vi "Defocus and Spherical Comp.vi"(1 "Spherical Step":dbl, 2 "Defocus Step":dbl, 3 "Step #":i32) -> ()   [LabVIEW 2014]
uses:
  DM_Dual_V2/Controls/Standard Action.ctl
panel:
  out "Map 2":dbl[][](graph)
  out "map 1":dbl[][](graph)
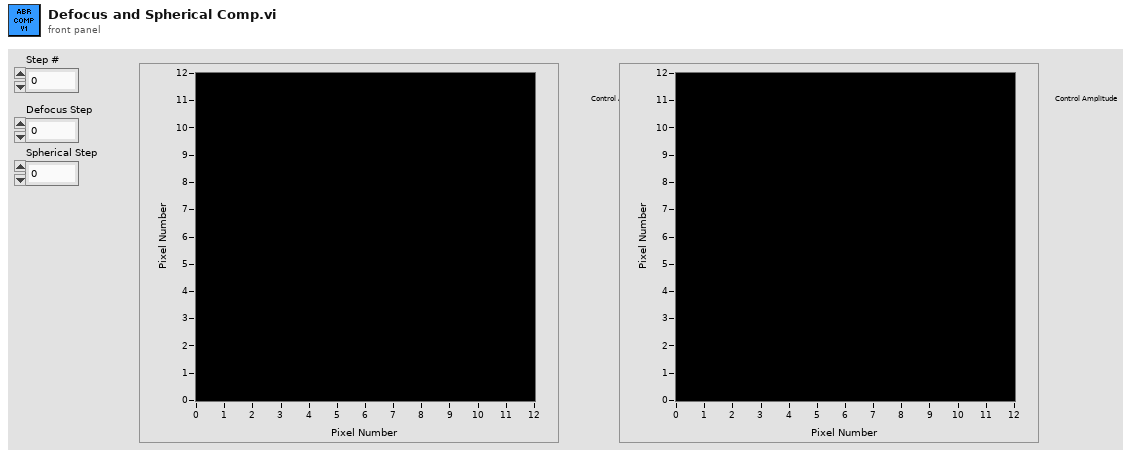
[diagram p1: front panel]
types:
  T1 = typedef "Standard Action.ctl" = enum16{"Read", "Write"}
  T2 = typedef "MirrorModes_DUAL.ctl" = cluster{"Mode":string, "Amplitude":dbl}[][]
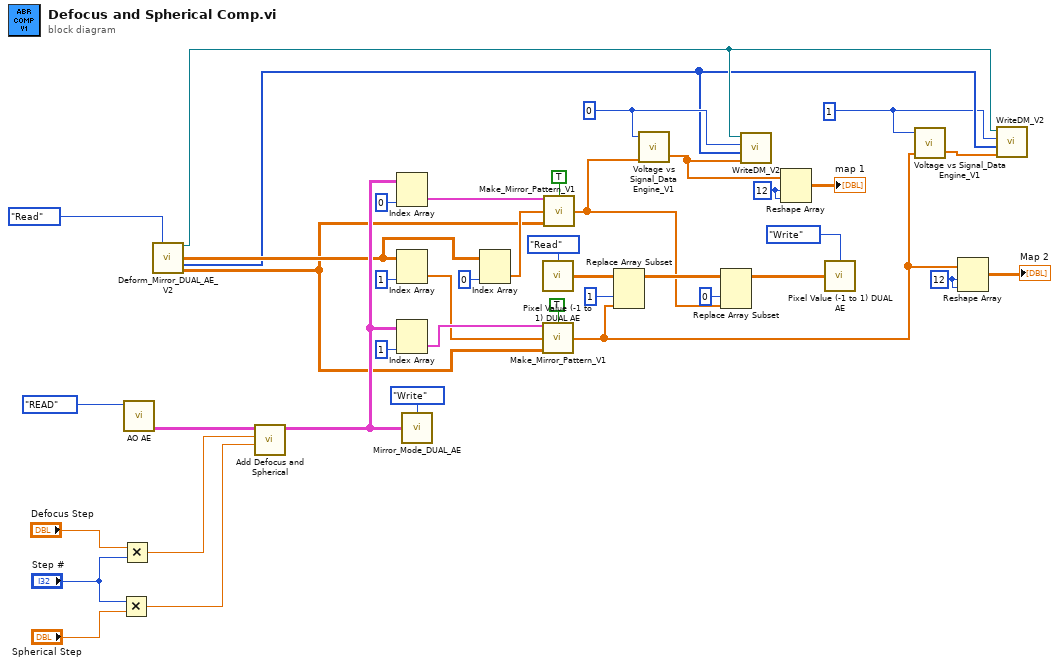
[diagram p0: block diagram]
diagram:
  w6 = 12 ("dimension size")
  w9 = 12 ("dimension size")
  w23 = 1 ("disabled index (col)")
  w27 = 0 ("disabled index (col)")
  n1 = Multiply(x="Step #", y="Spherical Step") -> (x*y=w18:dbl)
  n2 = Multiply(x="Defocus Step", y="Step #") -> (x*y=w19:dbl)
  n3 = call "AO AE.vi"("Action"=enum16{"READ", "WRITE"}."READ") -> ("Mirror Modes Out"=w1:T2)  [unwired: 8 in, 2 out]
  n4 = call "Deform_Mirror_DUAL_AE_V2.vi"("Action"=Standard_Action."Read") -> ("Refnum Out"=w25:refnum<k7>, "Flat Files Out"=w36:dbl[][], "Multi Map Data Out"=w24:i32[], "Mode Matrix Out"=w28:dbl[][][])  [unwired: 10 in, 1 out]
  n5 = call "Add Defocus and Spherical.vi"("Spherical Comp"=w18, "Defocus Comp"=w19, "Mirror Modes in"=w1) -> ("Mirror Modes out"=w39:T2)  [unwired: 8 in]
  n6 = Index Array(array=w39, index (col)=0 ("disabled index (col)")) -> (element=w30:cluster{"Mode":string, "Amplitude":dbl}[])  [unwired: 1 in]
  n7 = Index Array(array=w36, index (col)=1 ("disabled index (col)")) -> (element=w32:dbl[])  [unwired: 1 in]
  n8 = Index Array(array=w39, index (col)=1 ("disabled index (col)")) -> (element=w34:cluster{"Mode":string, "Amplitude":dbl}[])  [unwired: 1 in]
  n9 = call "Mirror_Mode_DUAL_AE.vi"("Action"=Standard_Action."Write", "Mirror Modes In"=w39) -> ()  [unwired: 13 in, 1 out]
  n10 = Index Array(array=w36, index (col)=0 ("disabled index (col)")) -> (element=w29:dbl[])  [unwired: 1 in]
  n11 = call "Pixel Value (-1 to 1) DUAL AE.vi"("Action"=Standard_Action."Read") -> ("Pixel Value (-1 to 1) Out"=w15:dbl[][])  [unwired: 14 in]
  n12 = call "Make_Mirror_Pattern_V1.vi"("Mirror Modes In"=w34, "Flat On?"=TRUE, "Flat File In"=w32, "Mirror Modes Array"=w28) -> ("Pixel Value U (-1 to 1)"=w5:dbl[])  [unwired: 11 in]
  n13 = call "Make_Mirror_Pattern_V1.vi"("Mirror Modes In"=w30, "Flat On?"=TRUE, "Flat File In"=w29, "Mirror Modes Array"=w28) -> ("Pixel Value U (-1 to 1)"=w11:dbl[])  [unwired: 11 in]
  n14 = Replace Array Subset(array=w15, new element=w5, index (col)=1 ("disabled index (col)")) -> (w13:dbl[][])  [unwired: 1 in]
  n15 = call "Voltage vs Signal_Data Engine_V1.vi"("Control Signal In (-1~1)"=w11, "DM #"=w27) -> ("Voltage Out (0~Max. Vol.)"=w8:dbl[])  [unwired: 1 in, 1 out]
  n16 = Replace Array Subset(array=w13, new element=w11, index (col)=0 ("disabled index (col)")) -> (w10:dbl[][])  [unwired: 1 in]
  n17 = call "WriteDM_V2.vi"("reference in"=w25, "nDevId"=w27, "MultiDM  Mapping"=w24, "Voltage Array in"=w8) -> ()  [unwired: 2 in, 2 out]
  n18 = Reshape Array(w8, w9, w9) -> (→"map 1":dbl[][])
  n19 = call "Pixel Value (-1 to 1) DUAL AE.vi"("Action"=Standard_Action."Write", "Pixel Value (-1 to 1)"=w10) -> ()  [unwired: 13 in, 1 out]
  n20 = call "Voltage vs Signal_Data Engine_V1.vi"("Control Signal In (-1~1)"=w5, "DM #"=w23) -> ("Voltage Out (0~Max. Vol.)"=w26:dbl[])  [unwired: 1 in, 1 out]
  n21 = Reshape Array(w5, w6, w6) -> (→"Map 2":dbl[][])
  n22 = call "WriteDM_V2.vi"("reference in"=w25, "nDevId"=w23, "MultiDM  Mapping"=w24, "Voltage Array in"=w26) -> ()  [unwired: 2 in, 2 out]
